vi "Begin.vi"(8 "error in (no error)":errorcluster, 11 "Configuration File in":refnum<class "Configuration File.lvclass">) -> (0 "error out":errorcluster, 3 "Configuration File out":refnum<class "Configuration File.lvclass">)   [LabVIEW 2018, in "Configuration File.lvlib" / "Configuration File.lvclass"]
doc: "This VI opens a configuration file in the robot."
uses:
  Configuration File.lvclass
  <vilib>/Utility/config.llb/Read Key (String).vi
  <vilib>/Rock Robotics/Network Tables/NT Write String.vi
  <vilib>/Utility/config.llb/NI_LVConfig.lvlib
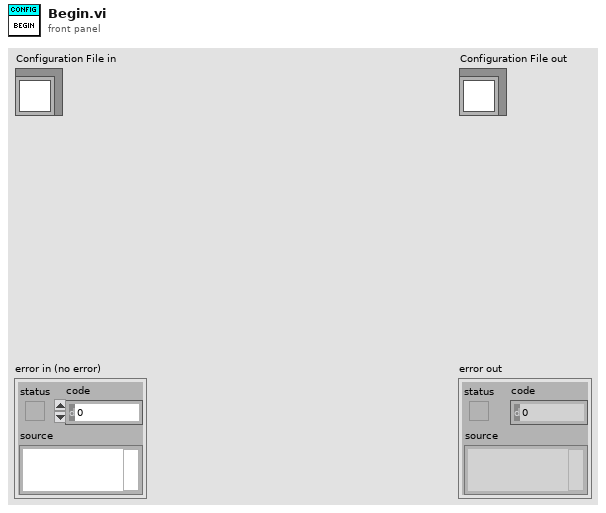
[diagram p1: front panel]
types:
  T1 = typedef "NI_LVConfig.lvlib/Config Data RefNum.ctl" = refnum<k1>
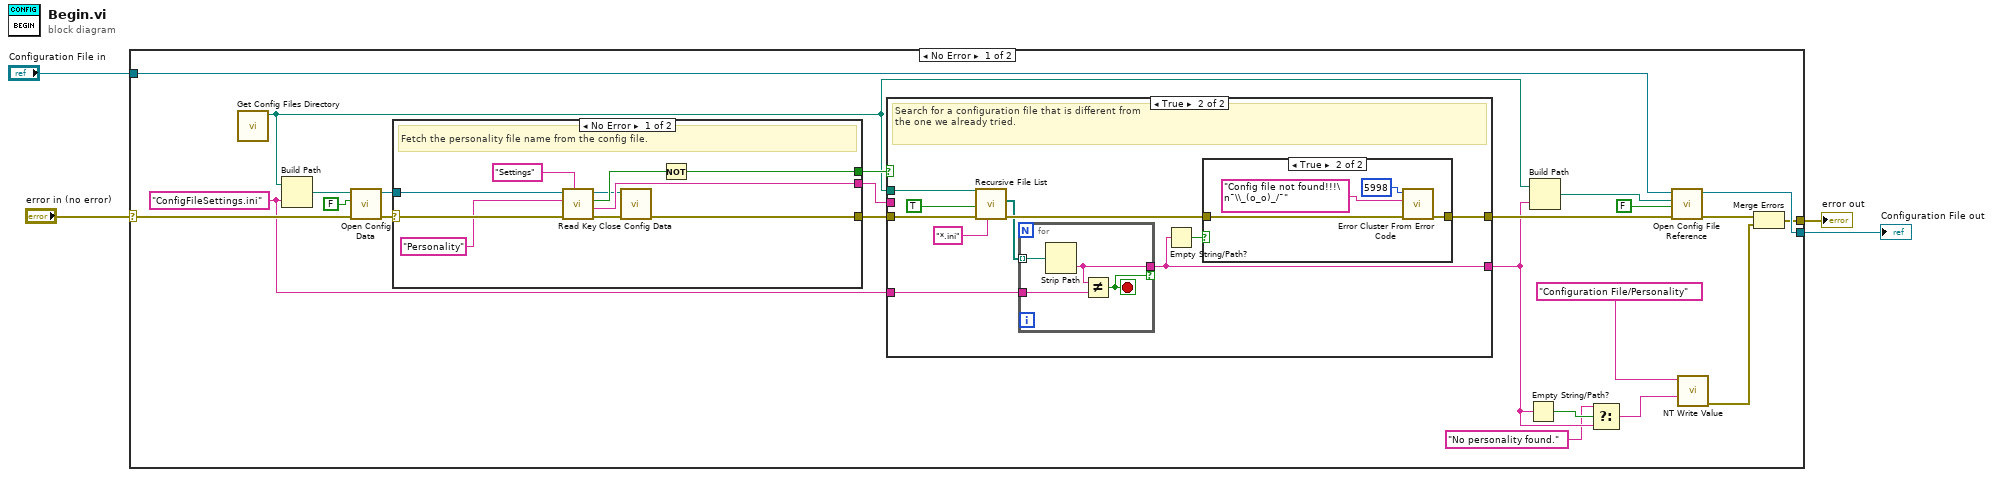
[diagram p0: block diagram]
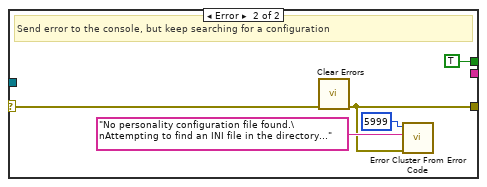
[diagram p4: hidden frame]
diagram:
  n1 = case shown="No Error" "error in (no error)" {
    selector: "error in (no error)" -> [w25 w65]
    tunnel: [w7 w65] -> w3
    tunnel: [w24 w64] -> w1
    tunnel: "Configuration File in" -> [w27 w64]
    frame No Error {
      w15 = "ConfigFileSettings.ini" ("name or relative path")
      n2 = call "Get Config Files Directory.vi"() -> ("configuration file path"=w14:path)  [unwired: 11 in]
      n3 = Build Path(base path=w14, name or relative path=w15) -> (appended path=w26:path)
      n4 = call <vilib>:"Open Config Data.vi"("error in (no error)"=w25, "create file if necessary (T)"=FALSE, "configuration file path"=w26) -> ("error out"=w21:errorcluster, "refnum"=w22:T1)  [unwired: 6 in, 1 out]
      n5 = case shown="No Error" w21 {
        selector: w21 -> [w57 w63]
        tunnel: w22 -> [w58 _]
        tunnel: [w54 _] -> w18
        tunnel: [w52 TRUE] -> w19
        tunnel: [w49 w59] -> w5
        frame No Error {
          # "Fetch the personality file name from the config file."
          n6 = call-poly <vilib>:"Read Key.vi"("section"="Settings", "error in (no error)"=w57, "key"="Personality", "refnum"=w58) -> ("error out"=w51:errorcluster, "value"=w54:string, "found?"=w53:bool, "refnum out"=w50:T1)  [unwired: 4 in]
          n7 = call <vilib>:"Close Config Data.vi"("error in (no error)"=w51, "refnum"=w50) -> ("error out"=w49:errorcluster)  [unwired: 8 in, 1 out]
          n8 = Not(x=w53) -> (.not. x?=w52:bool)
        }
        frame Error {
          # "Send error to the console, but keep searching for a configuration"
          n9 = call <vilib>:"Clear Errors.vi"("error in (no error)"=w63) -> ("error out"=w59:errorcluster)  [unwired: 5 in, 1 out]
          n10 = call <vilib>:"Error Cluster From Error Code.vi"("error in (no error)"=w59, "error message (\"\")"="No personality configuration file found.\nAttempting to find an INI file in the directory..." ("error message (\"\")"), "error code (0)"=5999) -> ()  [unwired: 6 in, 1 out]
        }
      }
      n11 = case shown="True" w19 {
        tunnel: w5 -> [w28 w39]
        tunnel: [w28 w31] -> w20
        tunnel: w14 -> [_ w37]
        tunnel: [w29 w34] -> w12
        tunnel: w18 -> [w29 _]
        tunnel: w15 -> [_ w32]
        frame False {
          # "Config file found, do nothing else."
        }
        frame True {
          # "Search for a configuration file that is different from\nthe one we already tried."
          n12 = call <vilib>:"Recursive File List.vi"("pattern"="*.ini", "error in (no error)"=w39, "Continue Recursing on Error? (F)"=TRUE, "Folder Path"=w37) -> ("error out"=w38:errorcluster, "All Files in Dir"=w33:path[])  [unwired: 3 in, 3 out]
          n13 = for {
            tunnel: [w47] -> w34 if=w45
            tunnel: w33 -> [w48] mode=indexing
            tunnel: w32 -> [w46]
            stop <- w45 stop-if-true
            n14 = Strip Path(path=w48) -> (name=w47:string)  [unwired: 1 out]
            n15 = Not Equal?(x=w47, y=w46) -> (x != y?=w45:bool)
          }
          n16 = Empty String/Path?(string/path=w34) -> (empty?=w30:bool)
          n17 = case shown="True" w30 {
            tunnel: w38 -> [w40 w44]
            tunnel: [w40 w43] -> w31
            frame False {
            }
            frame True {
              n18 = call <vilib>:"Error Cluster From Error Code.vi"("error in (no error)"=w44, "error message (\"\")"="Config file not found!!!\n¯\\_(o_o)_/¯" ("error message (\"\")"), "error code (0)"=5998) -> ("error out"=w43:errorcluster)  [unwired: 6 in]
            }
          }
        }
      }
      n19 = Empty String/Path?(string/path=w12) -> (empty?=w13:bool)
      n20 = Build Path(base path=w14, name or relative path=w12) -> (appended path=w17:path)
      n21 = Select(t="No personality found.", s=w13, f=w12) -> (s? t:f=w10:string)
      n22 = call "Open Config File Reference.vi"("error in (no error)"=w20, "create file if necessary (T)"=FALSE, "appended path"=w17, "Configuration File in"=w27) -> ("error out"=w8:errorcluster, "Configuration File out"=w24:refnum<class "Configuration File.lvclass">)  [unwired: 6 in]
      n23 = call-poly <vilib>:"NT Write Value.vi"("String"=w10, "Name"="Configuration File/Personality") -> ("error out"=w9:errorcluster)  [unwired: 9 in]
      n24 = Merge Errors(w8, w9) -> (w7:errorcluster)
    }
    frame Error {
    }
  }
  "error out" <- w3
  "Configuration File out" <- w1
